vi "SimpleMotorFF_Calculate_CalcAccel.vi"(9 "dT_Sec":dbl=0.02, 10 "VelSp":dbl, 11 "SIMPLE_MOTOR_FF":T1 {"KnInv" format="%13.4f"; "Ka" format="%13.4f"; "Kv" format="%13.4f"; "Ks" format="%13.4f"}) -> (3 "FeedForward":dbl)   [LabVIEW 2019, in "Trajectory_Library.lvlib"]
doc: "Calculates the feedforward from the gains and setpoints. Instead of Acceleration Setpoint being supplied as a setpoint, the acceleration is calculated based on the change in the Velocity setpoint.\n \nParameters:\n - SimpleMotorFF -- Data structure containing constants\n - velocity Setpoint -- The velocity setpoint. \n - dt -- The delta time (Seconds), default is 0.02 seconds.\nReturns:\n - FeedForward - The computed feedforward."
uses:
  Trajectory_Library.lvlib
  TypeDef/SIMPLE_MOTOR_FF.ctl
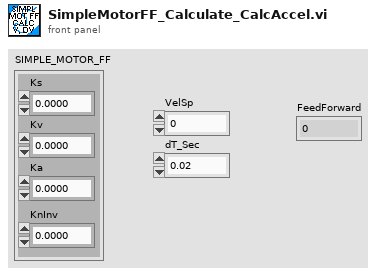
[diagram p1: front panel]
types:
  T1 = typedef "Trajectory_Library.lvlib/SIMPLE_MOTOR_FF.ctl" = cluster{"Ks":dbl, "Kv":dbl, "Ka":dbl, "KnInv":dbl}
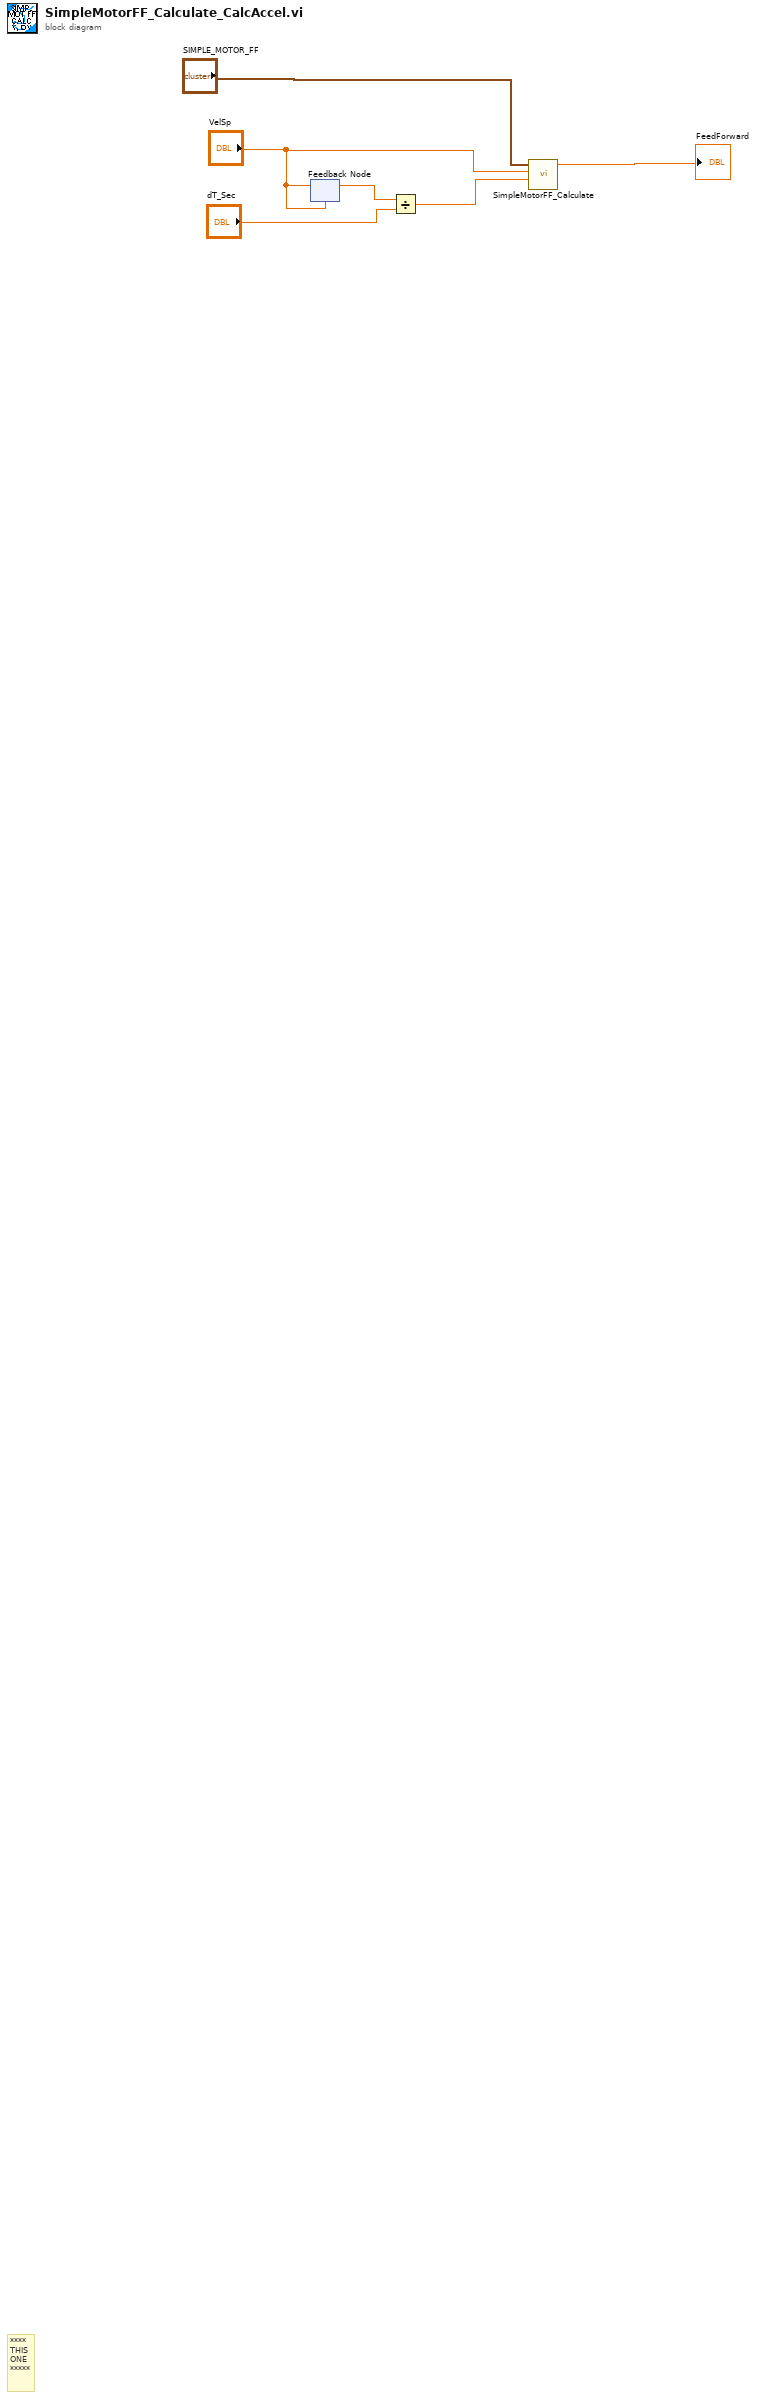
[diagram p0: block diagram]
diagram:
  # "****\nTHIS\nONE\n*****"
  n1 = feedback-in #1("VelSp") -> ()
  n2 = feedback #1("VelSp") -> (w3:dbl)
  n3 = Divide(x=w3, y="dT_Sec") -> (x/y=w1:dbl)
  n4 = call "SimpleMotorFF_Calculate.vi"("Accel"=w1, "Vel"="VelSp", "SIMPLE_MOTOR_FF"="SIMPLE_MOTOR_FF") -> ("FeedForward"=→"FeedForward":dbl)  [unwired: 8 in]
